vi "overlayCrosshairs.vi"(8 "error in":errorcluster, 11 "Image in":T1) -> (0 "error out":errorcluster, 3 "Image out":T1)   [LabVIEW 2015]
uses:
  <vilib>/vision/Image Controls.llb/IMAQ Image.ctl
panel:
  # "draw crosshairs"
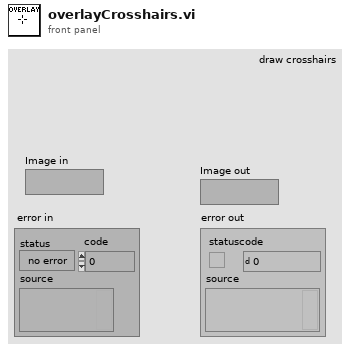
[diagram p1: front panel]
types:
  T1 = typedef "IMAQ Image.ctl" = refnum<image>
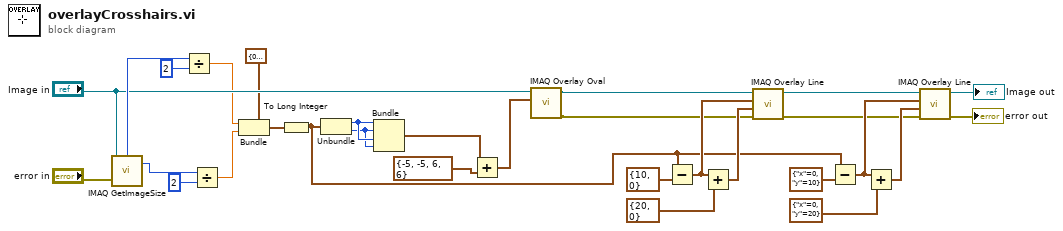
[diagram p0: block diagram]
diagram:
  n1 = call "IMAQ GetImageSize"("Image"="Image in", "error in (no error)"="error in") -> ("Y Resolution"=w28:i32, "X Resolution"=w30:i32)  [unwired: 2 in, 1 out]
  n2 = Divide(x=w30, y=2) -> (x/y=w10:dbl)
  n3 = Divide(x=w28, y=2) -> (x/y=w9:dbl)
  n4 = Bundle(cluster=cluster{"x":sgl, "y":sgl} {"x"=0.0, "y"=0.0} ("center 2"), "x"=w10, "y"=w9) -> (w5:cluster{"x":sgl, "y":sgl})
  n5 = To Long Integer(number=w5) -> (32bit integer=w3:cluster{"x":i32, "y":i32})
  n6 = Unbundle(w3) -> ("x"=w7:i32, "y"=w6:i32)
  n7 = Bundle("x"=w7, "y"=w6, "x"=w7, "y"=w6) -> (w4:cluster{"x":i32, "y":i32, "x":i32, "y":i32})  [unwired: 1 out]
  n8 = Add(x=w4, y=cluster{"y":i32, "x":i32, "y":i32, "x":i32} {"y"=-5, "x"=-5, "y"=6, "x"=6}) -> (x+y=w15:cluster{i32, i32, i32, i32})
  n9 = call "IMAQ Overlay Oval"("Bounding Rectangle"=w15, "Image"="Image in") -> ("error out"=w13:errorcluster, "Image Out"=w14:T1)  [unwired: 4 in, 4 out]
  n10 = Subtract(x=w3, y=cluster{"x":i32, "y":i32} {"x"=10, "y"=0}) -> (x-y=w24:cluster{"x":i32, "y":i32})
  n11 = Add(x=w24, y=cluster{"x":i32, "y":i32} {"x"=20, "y"=0}) -> (x+y=w22:cluster{"x":i32, "y":i32})
  n12 = call "IMAQ Overlay Line"("error in (no error)"=w13, "End Point"=w22, "Start Point"=w24, "Image"=w14) -> ("error out"=w16:errorcluster, "Image Out"=w17:T1)  [unwired: 2 in, 4 out]
  n13 = Subtract(x=w3, y=cluster{"x":i32, "y":i32} {"x"=0, "y"=10}) -> (x-y=w20:cluster{"x":i32, "y":i32})
  n14 = Add(x=w20, y=cluster{"x":i32, "y":i32} {"x"=0, "y"=20}) -> (x+y=w21:cluster{"x":i32, "y":i32})
  n15 = call "IMAQ Overlay Line"("error in (no error)"=w16, "End Point"=w21, "Start Point"=w20, "Image"=w17) -> ("error out"=→"error out":errorcluster, "Image Out"=→"Image out":T1)  [unwired: 2 in, 4 out]
